vi "Write_ControllerTimeout.vi"(8 "error in (no error)":errorcluster, 10 "ControlTimeout":i32, 11 "SubsystemData in":refnum<class "SubsystemData.lvclass">) -> (0 "error out":errorcluster, 3 "SubsystemData out":refnum<class "SubsystemData.lvclass">)   [LabVIEW 2017]
uses:
  SubsystemData.lvclass
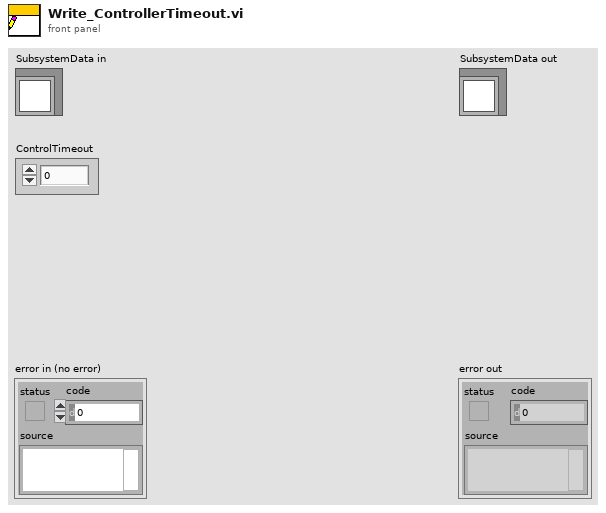
[diagram p1: front panel]
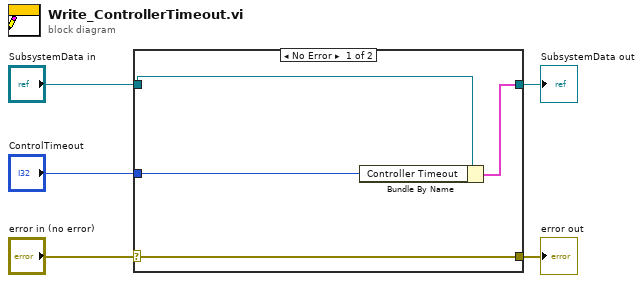
[diagram p0: block diagram]
diagram:
  n1 = case shown="No Error" "error in (no error)" {
    selector: "error in (no error)" -> [w9 w10]
    tunnel: [w9 w10] -> w4
    tunnel: [w7 w11] -> w2
    tunnel: "SubsystemData in" -> [w8 w11]
    tunnel: "ControlTimeout" -> [w6 _]
    frame No Error {
      n2 = Bundle By Name(cluster=w8, "Controller Timeout"=w6) -> (w7:cluster{})
    }
    frame Error {
    }
  }
  "error out" <- w4
  "SubsystemData out" <- w2
